vi "Host_muPathSamplingFPGA13.vi"() -> ()   [LabVIEW 2017]
uses:
  <vilib>/Utility/file.llb/Read From Spreadsheet File (I64).vi
  <vilib>/FPGAPlugInAG/cRIO-9082/niLvFpga_Open_cRIO-9082.vi
  <vilib>/rvi/interface/common/dynamic/niFpgaDynamicAddResources.vi
  <vilib>/FPGAPlugInAG/Dynamic/niLvFpga_Reset_Dynamic.vi
  <vilib>/Utility/error.llb/Error Cluster From Error Code.vi
  <vilib>/rvi/errors/niLvFpgaAdjustHostInterfaceError.vi
  <vilib>/rvi/interface/common/niFpgaWaitOnOcc.vi
  <vilib>/FPGAPlugInAG/Dynamic/niLvFpga_Run_Dynamic.vi
  <vilib>/Utility/file.llb/Write To Spreadsheet File (DBL).vi
  <vilib>/rvi/interface/nirviOpenFPGA/nirviOpenFPGA.xnode
  FPGA Bitfiles/simpletest_FPGATarget_muPathSamplingFP_3R5yrib4luo.lvbitx
  muPathSamplingFPGA27.vi
  <vilib>/rvi/interface/nirviMethod/nirviMethod.xnode
  <vilib>/rvi/interface/nirviReadWriteControl/nirviReadWriteControl.xnode
  <vilib>/FPGAPlugInAG/Dynamic/niLvFpga_ConfigureFifo_Dynamic.vi
  <vilib>/rvi/errors/niLvFpgaMergeErrorWithErrorCode.vi
  <vilib>/rvi/interface/Simulation/niFpgaSimulationCallBeginRW.vi
  NiFpgaLv.dll
  <vilib>/FPGAPlugInAG/Dynamic/niLvFpga_WriteFifo_Dynamic.vi
  <vilib>/FPGAPlugInAG/Dynamic/niLvFpga_StartFifo_Dynamic.vi
  <vilib>/FPGAPlugInAG/Dynamic/niLvFpga_ReadFifo_Dynamic.vi
panel:
  out "stage":dbl=4.0
  out "z output":dbl=4.67938232421875
  out "y output":dbl=5.690643310546875
  out "x output":dbl=-2.256500244140625
  out "deflection":dbl=0.00335693359375
  out "z":dbl=-4.658050537109375
  out "y":dbl=4.685882568359375
  out "x":dbl=0.370574951171875
  out "Elements Remaining":u64
  in  "whole map scanning":bool
  in  "mask file path":path=path "C:/Users/AnderssonLab/Desktop/yufan/sample locations/backup_a_upathlocations_E.txt"
  in  "mu path file path":path=path "C:/Users/AnderssonLab/Desktop/yufan/sample locations/backup_l_upathlocations.txt"
  out "FINISH_SIGNAL":bool
  in  "background value":dbl=-3.0
  in  "read def threshold":dbl=0.5
  out "Topography":dbl[][](graph)
  out "Empty Elements Remaining":u32
  out "Actual Depth":u32=2048
  in  "MASTER STOP":bool
  in  "Count(uSec)":u32=1 caption="Data Write Count(uSec)"
  in  "initial image_y":u16=1
  in  "initial image_x":u16=1
  in  "Threshold":T1={"x threshold"=0.06500244140625, "y threshold"=0.06500244140625, "z threshold"=0.649993896484375, "deflection threshold"=0.029998779296875, "x_scan threshold"=0.035003662109375}
  in  "z control":T2={"SetPoint (V)"=-5.0, "I"=400.0, "P"=0.259765625, "Initial I (V)"=0.0, "Upper Limit (V)"=9.900000095367432, "Lower Limit (V)"=-9.900000095367432}
  in  "deflection control":T3={"SetPoint (V)"=0.0, "scanning I"=370.0, "scanning P"=0.005859375, "Initial I (V)"=0.0, "Upper Limit (V)"=9.900000095367432, "Lower Limit (V)"=-9.900000095367432, "approach I"=370.0, "approach P"=0.005859375}
  in  "x control":T4={"SetPoint (V)"=0.0, "scanning I"=1850.0, "scanning P"=0.341796875, "Initial I (V)"=0.0, "Upper Limit (V)"=9.900000095367432, "Lower Limit (V)"=-9.900000095367432, "move I"=750.0, "move P"=0.341796875}
  in  "y control":T5={"SetPoint (V)"=0.0, "scanning I"=950.0, "scanning P"=0.341796875, "Initial I (V)"=0.0, "Upper Limit (V)"=9.900000095367432, "Lower Limit (V)"=-9.900000095367432, "move I"=750.0, "move P"=0.341796875}
  in  "ImageToSample":T6={"image size_x"=512, "image size_y"=512, "sample start_x"=0.0, "sample start_y"=0.0, "sample end_x"=6.0, "sample end_y"=6.0}
  in  "Clock (uSec)":T7={"XY Clock (uSec)"=20.0, "Z Clock (uSec)"=3.0, "Stage Clock (uSec)"=400.0, "muPathUpdate Clock (uSec)"=37.0, "Sampling Clock (uSec)"=6500.0, "pixel segment"=1000}
  # "mu path"
  # "whole map"
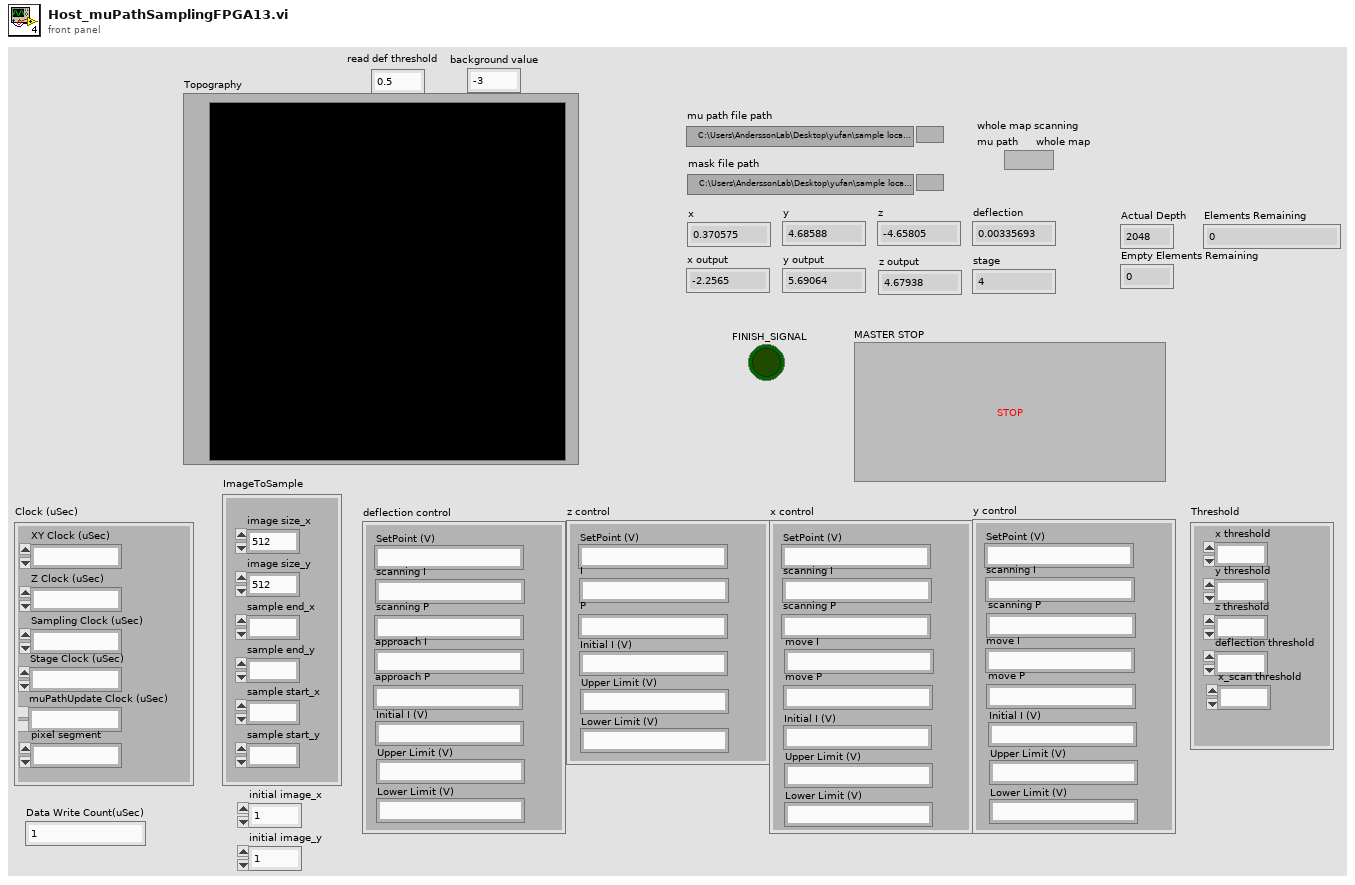
[diagram p1: front panel]
types:
  T1 = cluster{"x threshold":fxp<+/-,20,5>, "y threshold":fxp<+/-,20,5>, "z threshold":fxp<+/-,20,5>, "deflection threshold":fxp<+/-,20,5>, "x_scan threshold":fxp<+/-,20,5>}
  T2 = cluster{"SetPoint (V)":fxp<+/-,26,5>, "I":fxp<+,21,13>, "P":fxp<+,15,5>, "Initial I (V)":fxp<+/-,10,5>, "Upper Limit (V)":fxp<+/-,26,5>, "Lower Limit (V)":fxp<+/-,26,5>}
  T3 = cluster{"SetPoint (V)":fxp<+/-,26,5>, "scanning I":fxp<+,21,13>, "scanning P":fxp<+,15,5>, "Initial I (V)":fxp<+/-,10,5>, "Upper Limit (V)":fxp<+/-,26,5>, "Lower Limit (V)":fxp<+/-,26,5>, "approach I":fxp<+,21,13>, "approach P":fxp<+,15,5>}
  T4 = cluster{"SetPoint (V)":fxp<+/-,26,5>, "scanning I":fxp<+,21,13>, "scanning P":fxp<+,15,5>, "Initial I (V)":fxp<+/-,10,5>, "Upper Limit (V)":fxp<+/-,26,5>, "Lower Limit (V)":fxp<+/-,26,5>, "move I":fxp<+,21,13>, "move P":fxp<+/-,15,5>}
  T5 = cluster{"SetPoint (V)":fxp<+/-,26,5>, "scanning I":fxp<+,21,13>, "scanning P":fxp<+,15,5>, "Initial I (V)":fxp<+/-,10,5>, "Upper Limit (V)":fxp<+/-,26,5>, "Lower Limit (V)":fxp<+/-,26,5>, "move I":fxp<+,21,13>, "move P":fxp<+,15,5>}
  T6 = cluster{"image size_x":u16, "image size_y":u16, "sample start_x":fxp<+/-,26,5>, "sample start_y":fxp<+/-,26,5>, "sample end_x":fxp<+/-,26,5>, "sample end_y":fxp<+/-,26,5>}
  T7 = cluster{"XY Clock (uSec)":fxp<+,32,32>, "Z Clock (uSec)":fxp<+,32,32>, "Stage Clock (uSec)":fxp<+,32,32>, "muPathUpdate Clock (uSec)":fxp<+,32,32>, "Sampling Clock (uSec)":fxp<+,32,32>, "pixel segment":u32}
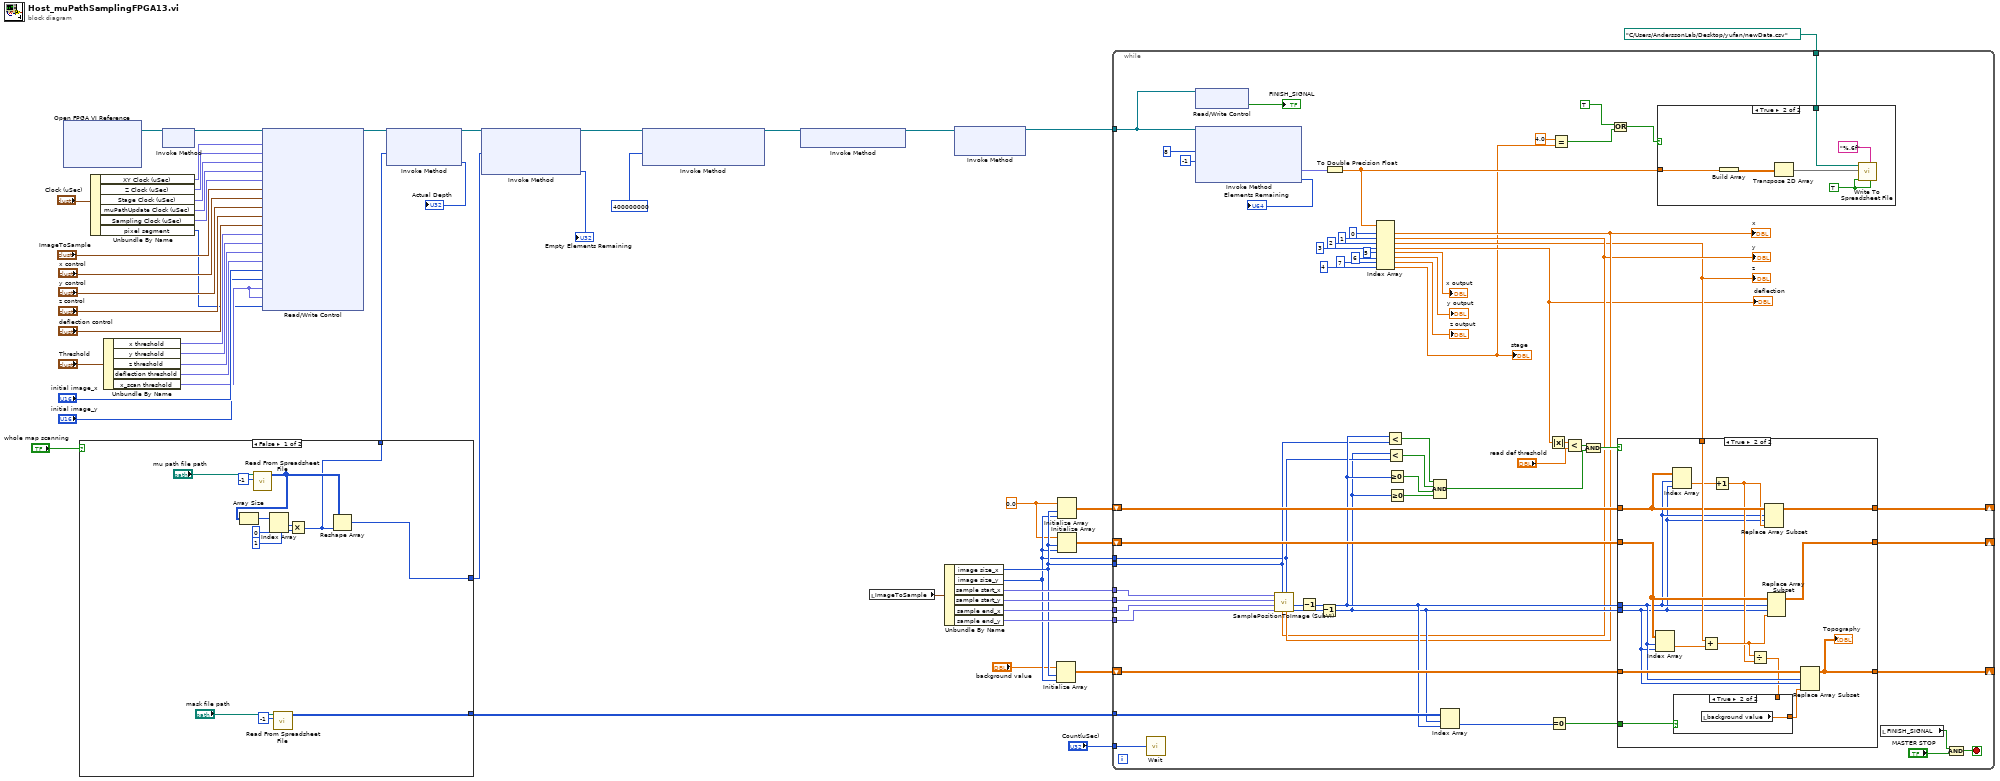
[diagram p0: block diagram]
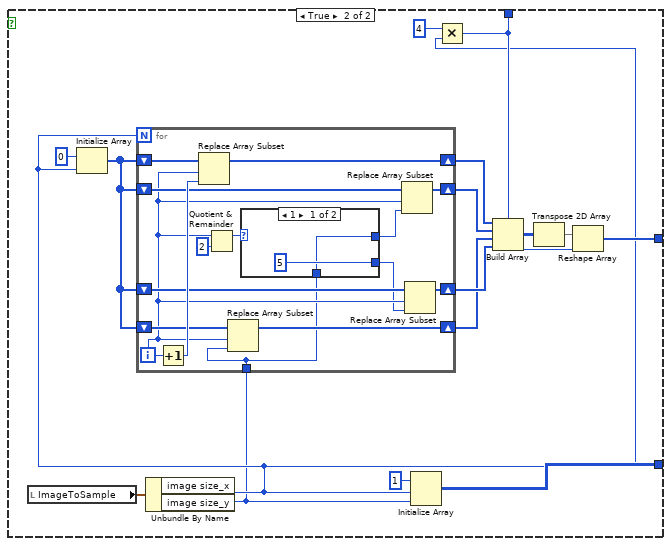
[diagram p2: hidden frame]
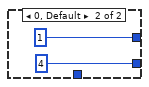
[diagram p3: hidden frame]
diagram:
  w9 = 0.0 ("element")
  n1 = xnode "Open FPGA VI Reference"() -> ("FPGA VI Reference Out"=w19:refnum<k20>)  [unwired: 2 in, 1 out]
  n2 = case shown="False" "whole map scanning" {
    tunnel: [w60 w78] -> w5
    tunnel: [w52 w65] -> w4
    tunnel: [w51 w66] -> w3
    frame False {
      n3 = call-poly <vilib>:"Read From Spreadsheet File.vi"("number of rows (all:-1)"=-1, "file path (dialog if empty)"="mu path file path") -> ("all rows"=w59:i64[][])  [unwired: 5 in, 4 out]
      n4 = Array Size(array=w59) -> (size(s)=w56:i32[])
      n5 = Index Array(array=w56, index #1=0 ("index"), index #2=1 ("index")) -> (element #1=w57:i32, element #2=w58:i32)
      n6 = call-poly <vilib>:"Read From Spreadsheet File.vi"("number of rows (all:-1)"=-1, "file path (dialog if empty)"="mask file path") -> ("all rows"=w60:i64[][])  [unwired: 5 in, 4 out]
      n7 = Multiply(x=w57, y=w58) -> (x*y=w51:i32)
      n8 = Reshape Array(w59, w51) -> (w52:i64[])
    }
    frame True {
      n9 = local read "ImageToSample"() -> (w76:T6)
      n10 = Unbundle By Name(w76) -> ("image size_x"=w64:u16, "image size_y"=w63:u16)
      n11 = Initialize Array(u32 0 ("element"), w64) -> (w68:u32[])
      n12 = for {
        N: w64 -> [_]
        shift-right: [w91] -> w72
        shift-left: w68 -> [w93]
        shift-right: [w89] -> w69
        shift-left: w68 -> [w90]
        shift-right: [w84] -> w70
        shift-left: w68 -> [w85]
        shift-right: [w83] -> w71
        shift-left: w68 -> [w82]
        tunnel: w63 -> [w79]
        i -> [w81]
        n13 = Increment(x=w81) -> (x+1=w92:i32)
        n14 = Replace Array Subset(array=w93, new element=w92, index=w81) -> (w91:u32[])
        n15 = Quotient & Remainder(x=w81, y=2) -> (x-y*floor(x/y)=w88:i32)  [unwired: 1 out]
        n16 = Replace Array Subset(array=w85, new element=w79, index=w81) -> (w84:u32[])
        n17 = case shown="1" w88 {
          tunnel: [w94 u32 1 ("new element/subarray")] -> w86
          tunnel: [u32 5 ("new element/subarray") u32 4 ("new element/subarray")] -> w80
          tunnel: w79 -> [w94 _]
          frame 1 {
          }
          frame 0, Default {
          }
        }
        n18 = Replace Array Subset(array=w90, new element=w86, index=w81) -> (w89:u32[])
        n19 = Replace Array Subset(array=w82, new element=w80, index=w81) -> (w83:u32[])
      }
      n20 = Initialize Array(u8 1 ("element"), w64, w63) -> (w78:u8[][])
      n21 = Multiply(x=u32 4, y=w64) -> (x*y=w66:u32)
      n22 = Build Array(w72, w69, w70, w71) -> (w73:u32[][])
      n23 = Transpose 2D Array(2D array=w73) -> (transposed array=w74:u32[][])
      n24 = Reshape Array(w74, w66) -> (w65:u32[])
    }
  }
  n25 = Unbundle By Name("Clock (uSec)") -> ("XY Clock (uSec)"=w46:fxp<+,32,32>, "Z Clock (uSec)"=w45:fxp<+,32,32>, "Stage Clock (uSec)"=w44:fxp<+,32,32>, "muPathUpdate Clock (uSec)"=w43:fxp<+,32,32>, "Sampling Clock (uSec)"=w42:fxp<+,32,32>, "pixel segment"=w2:u32)
  n26 = Unbundle By Name("Threshold") -> ("x threshold"=w35:fxp<+/-,20,5>, "y threshold"=w21:fxp<+/-,20,5>, "z threshold"=w34:fxp<+/-,20,5>, "deflection threshold"=w33:fxp<+/-,20,5>, "x_scan threshold"=w20:fxp<+/-,20,5>)
  n27 = xnode "Invoke Method"("FPGA VI Reference In"=w19) -> ("FPGA VI Reference Out"=w48:refnum<k20>)  [unwired: 1 in, 1 out]
  n28 = xnode "Read/Write Control"("FPGA VI Reference In"=w48, "XY Clock (uSec)"=w46, "Z Clock (uSec)"=w45, "Stage Clock (uSec)"=w44, "muPathUpdate Clock (uSec)"=w43, "Sampling Clock (uSec)"=w42, "ImageToSample"="ImageToSample", "x control"="x control", "y control"="y control", "z control"="z control", "deflection control"="deflection control", "x threshold"=w35, "y threshold"=w21, "z threshold"=w34, "deflection threshold"=w33, "initial image_x"="initial image_x", "initial image_y"="initial image_y", "x_scan threshold"=w20, "y_scan threshold"=w20, "pixel segment"=w2) -> ("FPGA VI Reference Out"=w24:refnum<k20>)  [unwired: 1 in, 1 out]
  n29 = xnode "Invoke Method"("FPGA VI Reference In"=w24, "Requested Depth"=w3) -> ("FPGA VI Reference Out"=w28:refnum<k20>, "Actual Depth"=→"Actual Depth":u32)  [unwired: 1 in, 1 out]
  n30 = xnode "Invoke Method"("FPGA VI Reference In"=w28, "Data"=w4) -> ("FPGA VI Reference Out"=w25:refnum<k20>, "Empty Elements Remaining"=→"Empty Elements Remaining":u32)  [unwired: 2 in, 1 out]
  n31 = xnode "Invoke Method"("FPGA VI Reference In"=w25, "Requested Depth"=u32 400000000) -> ("FPGA VI Reference Out"=w1:refnum<k20>)  [unwired: 1 in, 2 out]
  n32 = xnode "Invoke Method"("FPGA VI Reference In"=w1) -> ("FPGA VI Reference Out"=w23:refnum<k20>)  [unwired: 1 in, 1 out]
  n33 = local read "ImageToSample"() -> (w18:T6)
  n34 = Unbundle By Name(w18) -> ("image size_x"=w11:u16, "image size_y"=w10:u16, "sample start_x"=w17:fxp<+/-,26,5>, "sample start_y"=w16:fxp<+/-,26,5>, "sample end_x"=w15:fxp<+/-,26,5>, "sample end_y"=w14:fxp<+/-,26,5>)
  n35 = xnode "Invoke Method"("FPGA VI Reference In"=w23) -> ("FPGA VI Reference Out"=w22:refnum<k20>)  [unwired: 2 in, 1 out]
  n36 = Initialize Array("background value", w11, w10) -> (w8:dbl[][])
  n37 = Initialize Array(w9, w11, w10) -> (w13:dbl[][])
  n38 = Initialize Array(w9, w11, w10) -> (w12:dbl[][])
  n39 = while {
    tunnel: "Count(uSec)" -> [w157]
    tunnel: w22 -> [w123]
    tunnel: path "C:/Users/AnderssonLab/Desktop/yufan/newData.csv" ("file path (dialog if empty)") -> [w156]
    tunnel: w11 -> [w137]
    tunnel: w10 -> [w136]
    tunnel: w17 -> [w153]
    tunnel: w16 -> [w152]
    tunnel: w15 -> [w151]
    tunnel: w14 -> [w150]
    shift-right: [w146] -> _
    shift-left: w13 -> [w147]
    shift-right: [w144] -> _
    shift-left: w12 -> [w145]
    shift-right: [w142] -> _
    shift-left: w8 -> [w143]
    tunnel: w5 -> [w141]
    stop <- w126 stop-if-true
    n40 = call "Wait"("Count(uSec)"=w157) -> ()  [unwired: 1 out]
    n41 = xnode "Read/Write Control"("FPGA VI Reference In"=w123) -> ("signalToStop"=→"FINISH_SIGNAL":bool)  [unwired: 1 in, 2 out]
    n42 = xnode "Invoke Method"("FPGA VI Reference In"=w123, "Number of Elements"=u32 8, "Timeout (ms)"=-1) -> ("Data"=w119:fxp<+/-,25,5>[], "Elements Remaining"=→"Elements Remaining":u32)  [unwired: 1 in, 2 out]
    n43 = To Double Precision Float(number=w119) -> (double precision float=w118:dbl[])
    n44 = Index Array(array=w118, index #1=0 ("index"), index #2=1 ("index"), index #3=2 ("index"), index #4=3 ("index"), index #5=5 ("index"), index #6=6 ("index"), index #7=7 ("index"), index #8=4 ("index")) -> (element #1=w110:dbl, element #2=w109:dbl, element #3=w108:dbl, element #4=w107:dbl, element #5=→"x output":dbl, element #6=→"y output":dbl, element #7=→"z output":dbl, element #8=w101:dbl)
    "x" <- w110
    "y" <- w109
    "z" <- w108
    "deflection" <- w107
    "stage" <- w101
    n45 = call "SamplePositionToImage (SubVI).vi"("sample_y"=w110, "image size_y"=w136, "sample_x"=w109, "image size_x"=w137, "sample end_y"=w150, "sample end_x"=w151, "sample start_y"=w152, "sample start_x"=w153) -> ("image_y"=w148:u16, "image_x"=w149:u16)  [unwired: 2 out]
    n46 = Decrement(x=w149) -> (x-1=w138:u16)
    n47 = Decrement(x=w148) -> (x-1=w135:u16)
    n48 = Less?(x=w138, y=w137) -> (x < y?=w132:bool)
    n49 = Less?(x=w135, y=w136) -> (x < y?=w131:bool)
    n50 = Greater Or Equal To 0?(x=w138) -> (x >= 0?=w130:bool)
    n51 = Greater Or Equal To 0?(x=w135) -> (x >= 0?=w129:bool)
    n52 = Compound Arithmetic op=AND(w132, w131, w130, w129) -> (w128:bool)
    n53 = Index Array(array=w141, index (row)=w135, index (col)=w138) -> (element=w140:i64)
    n54 = Absolute Value(x=w107) -> (abs(x)=w155:dbl)
    n55 = Equal To 0?(x=w140) -> (x = 0?=w139:bool)
    n56 = Equal?(x=4.0, y=w101) -> (x = y?=w98:bool)
    n57 = Less?(x=w155, y="read def threshold") -> (x < y?=w134:bool)
    n58 = And(x=w134, y=w128) -> (x .and. y?=w133:bool)
    n59 = Or(x=TRUE, y=w98) -> (x .or. y?=w99:bool)
    n60 = case shown="True" w133 {
      tunnel: w147 -> [w166 w179]
      tunnel: [w166 w177] -> w146
      tunnel: w145 -> [w165 w182]
      tunnel: [w165 w176] -> w144
      tunnel: w138 -> [_ w172]
      tunnel: w135 -> [_ w171]
      tunnel: w108 -> [_ w180]
      tunnel: w143 -> [w164 w173]
      tunnel: [w164 w170] -> w142
      tunnel: w139 -> [_ w169]
      frame False {
      }
      frame True {
        n61 = Index Array(array=w182, index (row)=w172, index (col)=w171) -> (element=w181:dbl)
        n62 = Index Array(array=w179, index (row)=w172, index (col)=w171) -> (element=w178:dbl)
        n63 = Add(x=w180, y=w181) -> (x+y=w175:dbl)
        n64 = Increment(x=w178) -> (x+1=w174:dbl)
        n65 = Divide(x=w175, y=w174) -> (x/y=w167:dbl)
        n66 = case shown="True" w169 {
          tunnel: [w183 w184] -> w168
          tunnel: w167 -> [w183 _]
          frame False {
          }
          frame True {
            n67 = local read "background value"() -> (w184:dbl)
          }
        }
        n68 = Replace Array Subset(array=w179, new element=w174, index (row)=w172, index (col)=w171) -> (w177:dbl[][])
        n69 = Replace Array Subset(array=w182, new element=w175, index (row)=w172, index (col)=w171) -> (w176:dbl[][])
        n70 = Replace Array Subset(array=w173, new element=w168, index (row)=w172, index (col)=w171) -> (w170:dbl[][])
        "Topography" <- w170
      }
    }
    n71 = case shown="True" w99 {
      tunnel: w156 -> [_ w161]
      tunnel: w118 -> [_ w158]
      frame False {
      }
      frame True {
        w163 = TRUE
        n72 = Build Array(w158) -> (w160:dbl[][])
        n73 = Transpose 2D Array(2D array=w160) -> (transposed array=w159:dbl[][])
        n74 = call-poly <vilib>:"Write To Spreadsheet File.vi"("transpose? (no:F)"=w163, "format (%.3f)"="%.6f", "append to file? (new file:F)"=w163, "2D data"=w159, "file path (dialog if empty)"=w161) -> ()  [unwired: 3 in, 1 out]
      }
    }
    n75 = local read "FINISH_SIGNAL"() -> (w124:bool)
    n76 = And(x=w124, y="MASTER STOP") -> (x .and. y?=w126:bool)
  }
